vi "Values.vi"(8 "error in (no error)":errorcluster, 11 "Array In":refnum<class "Array.lvclass">) -> (0 "error out":errorcluster, 1 "Values":refnum<class>[](array[class]), 3 "Array Out":refnum<class "Array.lvclass">)   [LabVIEW 2013, in "LapDog.Collections.v1.Maps.Implementations.lvlib" / "Array.lvclass"]
doc: "Returns a copy of all values in the map."
uses:
  Array.lvclass
  Array.lvclass/Array.ctl
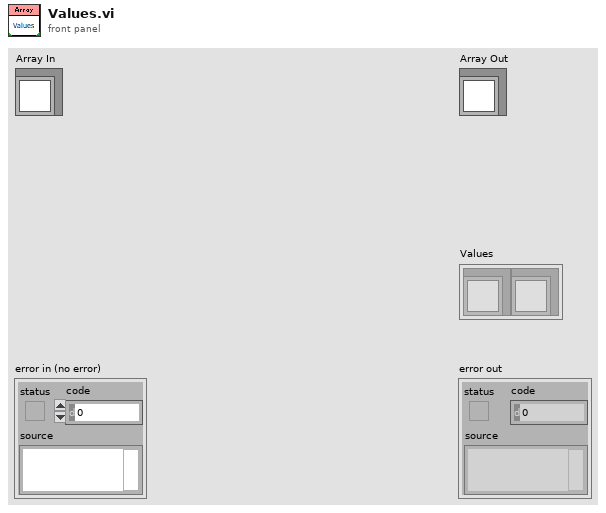
[diagram p1: front panel]
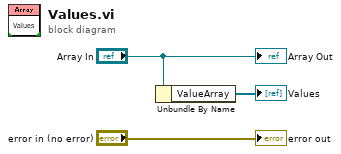
[diagram p0: block diagram]
diagram:
  n1 = Unbundle By Name("Array In") -> ("ValueArray"=→"Values":refnum<class>[])
  "error out" <- "error in (no error)"
  "Array Out" <- "Array In"
